vi "probe pulse.vi"(0 "Absolute start time (ms)":dbl=62793.546 format="%.3f", 1 "Static input":T4(array[cluster])=[{"Times"=[954.0, 1000.1, 6500.0], "Voltages"=[-0.05, -0.95, 2.0], "Enable Ch"=TRUE, "Hinge Points"=3}, {"Times"=[944.0, 994.0, 1000.0], "Voltages"=[-1.0, 1.65, -1.0], "Enable Ch"=TRUE, "Hinge Points"=3}, {"Times"=[944.0, 994.0, 1000.0], "Voltages"=[0.0, 0.4, -1.0], "Enable Ch"=TRUE, "Hinge Points"=3}, {"Times"=[944.0, 994.0, 1000.0], "Voltages"=[4.0, 0.65, -1.0], "Enable Ch"=TRUE, "Hinge Points"=3}, {"Times"=[992.0, 1000.6, 62293.246, 62294.046], "Voltages"=[0.0, 2.7, -0.8, 0.0], "Enable Ch"=TRUE, "Hinge Points"=4}, {"Times"=[1000.6, 1011.1], "Voltages"=[0.3, 3.0], "Enable Ch"=TRUE, "Hinge Points"=2}, {"Times"=[], "Voltages"=[], "Enable Ch"=TRUE, "Hinge Points"=0}, {"Times"=[62288.546], "Voltages"=[0.0], "Enable Ch"=TRUE, "Hinge Points"=1}, {"Times"=[944.0, 994.0, 1000.1, 1004.1, 6500.0], "Voltages"=[0.1635, 0.04, -0.625, 0.0, 1.0], "Enable Ch"=TRUE, "Hinge Points"=5}, {"Times"=[994.0, 1000.0, 1001.0, 1003.1, 1203.1, 1208.1, 1213.1, 1218.1, 1223.1, 1228.1, 1233.1, 1238.1, 1243.1, 1248.1, 1253.1, 1258.1, 1263.1, 1268.1, 1273.1, 1278.1, 1283.1, 1288.1, 1293.1, 1298.1, 1303.1, 1308.1, 1313.1, 1318.1, 1323.1, 1328.1, 1333.1, 1338.1, 1343.1, 1348.1, 1353.1, 1358.1, 1363.1, 1368.1, 1373.1, 1378.1, 1383.1, 1388.1, 1393.1, 1398.1, 1403.1, 1408.1, 1413.1, 1418.1, 1423.1, 1428.1, 1433.1, 1438.1, 1443.1, 1448.1, 1453.1, 1458.1, 1463.1, 1468.1, 1473.1, 1478.1, 1483.1, 1488.1, 1493.1, 1498.1, 1503.1, 1508.1, 1513.1, 1518.1, 1523.1, 1528.1, 1533.1, 1538.1, 1543.1, 1548.1, 1553.1, 1558.1, 1563.1, 1568.1, 1573.1, 1578.1, 1583.1, 1588.1, 1593.1, 1598.1, 1603.1, 1608.1, 1613.1, 1618.1, 1623.1, 1628.1, 1633.1, 1638.1, 1643.1, 1648.1, 1653.1, 1658.1, 1663.1, 1668.1, 1673.1, 1678.1, 1683.1, 1688.1, 1693.1, 1698.1, 1703.1, 5499.9], "Voltages"=[-1.0, -10.0, 0.0, 1.8, 1.8, 1.844, 1.8880000000000001, 1.932, 1.976, 2.02, 2.064, 2.108, 2.152, 2.196, 2.24, 2.2840000000000003, 2.3280000000000003, 2.372, 2.4160000000000004, 2.46, 2.504, 2.548, 2.592, 2.636, 2.68, 2.724, 2.7680000000000002, 2.8120000000000003, 2.856, 2.9000000000000004, 2.944, 2.9880000000000004, 3.032, 3.076, 3.12, 3.164, 3.208, 3.2520000000000002, 3.2960000000000003, 3.3400000000000003, 3.3840000000000003, 3.428, 3.4720000000000004, 3.516, 3.5600000000000005, 3.604, 3.648, 3.692, 3.736, 3.7800000000000002, 3.824, 3.8680000000000003, 3.912, 3.9560000000000004, 4.0, 4.0440000000000005, 4.088, 4.132000000000001, 4.176, 4.220000000000001, 4.264, 4.308000000000001, 4.352, 4.396, 4.44, 4.484, 4.5280000000000005, 4.572, 4.6160000000000005, 4.66, 4.704000000000001, 4.748, 4.792000000000001, 4.836, 4.880000000000001, 4.924, 4.968, 5.0120000000000005, 5.056, 5.1000000000000005, 5.144, 5.188000000000001, 5.232, 5.276000000000001, 5.32, 5.364000000000001, 5.408, 5.452000000000001, 5.496, 5.54, 5.5840000000000005, 5.628, 5.672000000000001, 5.716, 5.760000000000001, 5.804, 5.848, 5.892, 5.936, 5.98, 6.024, 6.0680000000000005, 6.112, 6.156000000000001, 6.2, -1.0], "Enable Ch"=TRUE, "Hinge Points"=106}, {"Times"=[1001.0, 978.1, 1008.1, 1183.1, 1188.1, 1193.1, 1198.1, 1203.1, 1208.1, 1213.1, 1218.1, 1223.1, 1228.1, 1233.1, 1238.1, 1243.1, 1248.1, 1253.1, 1258.1, 1263.1, 1268.1, 1273.1, 1278.1, 1283.1, 1288.1, 1293.1, 1298.1, 1303.1, 1308.1, 1313.1, 1318.1, 1323.1, 1328.1, 1333.1, 1338.1, 1343.1, 1348.1, 1353.1, 1358.1, 1363.1, 1368.1, 1373.1, 1378.1, 1383.1, 1388.1, 1393.1, 1398.1, 1403.1, 1408.1, 1413.1, 1418.1, 1423.1, 1428.1, 1433.1, 1438.1, 1443.1, 1448.1, 1453.1, 1458.1, 1463.1, 1468.1, 1473.1, 1478.1, 1483.1, 1488.1, 1493.1, 1498.1, 1503.1, 1508.1, 1513.1, 1518.1, 1523.1, 1528.1, 1533.1, 1538.1, 1543.1, 1548.1, 1553.1, 1558.1, 1563.1, 1568.1, 1573.1, 1578.1, 1583.1, 1588.1, 1593.1, 1598.1, 1603.1, 1608.1, 1613.1, 1618.1, 1623.1, 1628.1, 1633.1, 1638.1, 1643.1, 1648.1, 1653.1, 1658.1, 1663.1, 1668.1, 1673.1, 1678.1, 1683.1, 5505.0, 62273.546], "Voltages"=[-0.4, -2.5, -0.78, -0.78, -0.7989, -0.8178000000000001, -0.8367, -0.8556, -0.8745, -0.8934, -0.9123, -0.9312, -0.9501000000000001, -0.9690000000000001, -0.9879, -1.0068000000000001, -1.0257, -1.0446, -1.0635, -1.0824, -1.1013000000000002, -1.1202, -1.1391, -1.158, -1.1769, -1.1958, -1.2147000000000001, -1.2336, -1.2525, -1.2714, -1.2903, -1.3092000000000001, -1.3281, -1.347, -1.3659, -1.3848, -1.4037000000000002, -1.4226, -1.4415, -1.4604, -1.4793, -1.4982, -1.5171000000000001, -1.536, -1.5549, -1.5738, -1.5927, -1.6116000000000001, -1.6305, -1.6494, -1.6683, -1.6872, -1.7061000000000002, -1.725, -1.7439, -1.7628, -1.7817, -1.8006, -1.8195000000000001, -1.8384, -1.8573, -1.8762, -1.8951, -1.914, -1.9329, -1.9518, -1.9707000000000001, -1.9896, -2.0084999999999997, -2.0274, -2.0463, -2.0652, -2.0841000000000003, -2.1029999999999998, -2.1219, -2.1408, -2.1597, -2.1786000000000003, -2.1975, -2.2164, -2.2353, -2.2542, -2.2731000000000003, -2.292, -2.3109, -2.3298, -2.3487, -2.3676000000000004, -2.3865, -2.4054, -2.4243, -2.4432, -2.4621, -2.481, -2.4999000000000002, -2.5187999999999997, -2.5377, -2.5566, -2.5755, -2.5944000000000003, -2.6132999999999997, -2.6322, -2.6511, -2.67, -1.5, -1.5], "Enable Ch"=TRUE, "Hinge Points"=106}, {"Times"=[944.0, 994.0, 1000.6, 62291.546, 62294.046], "Voltages"=[0.15, 0.2, 2.5, -0.4, 0.0], "Enable Ch"=TRUE, "Hinge Points"=5}, {"Times"=[5500.0, 62273.546, 62273.548, 62273.55, 62273.552, 62273.554000000004, 62273.556000000004, 62273.558000000005, 62273.560000000005, 62273.562000000005, 62273.564, 62273.566, 62273.568, 62273.57, 62273.572, 62273.574, 62273.576, 62273.578, 62273.58, 62273.582, 62273.584, 62273.586], "Voltages"=[2.98, 2.98, 2.826, 2.672, 2.518, 2.364, 2.21, 2.056, 1.902, 1.748, 1.594, 1.44, 1.286, 1.1320000000000001, 0.9780000000000002, 0.8239999999999998, 0.6699999999999999, 0.516, 0.3620000000000001, 0.20800000000000018, 0.053999999999999826, -0.10000000000000009], "Enable Ch"=TRUE, "Hinge Points"=22}, {"Times"=[5500.0, 5600.0, 5609.0, 5618.0, 5627.0, 5636.0, 5645.0, 5654.0, 5663.0, 5672.0, 5681.0, 5690.0, 5699.0, 5708.0, 5717.0, 5726.0, 5735.0, 5744.0, 5753.0, 5762.0, 5771.0, 5780.0, 5789.0, 5798.0, 5807.0, 5816.0, 5825.0, 5834.0, 5843.0, 5852.0, 5861.0, 5870.0, 5879.0, 5888.0, 5897.0, 5906.0, 5915.0, 5924.0, 5933.0, 5942.0, 5951.0, 5960.0, 5969.0, 5978.0, 5987.0, 5996.0, 6005.0, 6014.0, 6023.0, 6032.0, 6041.0, 6050.0, 6059.0, 6068.0, 6077.0, 6086.0, 6095.0, 6104.0, 6113.0, 6122.0, 6131.0, 6140.0, 6149.0, 6158.0, 6167.0, 6176.0, 6185.0, 6194.0, 6203.0, 6212.0, 6221.0, 6230.0, 6239.0, 6248.0, 6257.0, 6266.0, 6275.0, 6284.0, 6293.0, 6302.0, 6311.0, 6320.0, 6329.0, 6338.0, 6347.0, 6356.0, 6365.0, 6374.0, 6383.0, 6392.0, 6401.0, 6410.0, 6419.0, 6428.0, 6437.0, 6446.0, 6455.0, 6464.0, 6473.0, 6482.0, 6491.0, 6500.0, 62273.546, 62303.546], "Voltages"=[0.5, 0.5, 0.5067, 0.5134, 0.5201, 0.5268, 0.5335, 0.5402, 0.5468999999999999, 0.5536, 0.5603, 0.567, 0.5737, 0.5804, 0.5871, 0.5938, 0.6005, 0.6072, 0.6139, 0.6206, 0.6273, 0.634, 0.6407, 0.6474, 0.6541, 0.6608, 0.6675, 0.6742, 0.6809, 0.6876, 0.6942999999999999, 0.701, 0.7077, 0.7143999999999999, 0.7211, 0.7278, 0.7344999999999999, 0.7412, 0.7479, 0.7545999999999999, 0.7613, 0.768, 0.7746999999999999, 0.7814, 0.7881, 0.7948, 0.8015, 0.8082, 0.8149, 0.8216, 0.8283, 0.835, 0.8416999999999999, 0.8484, 0.8551, 0.8617999999999999, 0.8684999999999999, 0.8752, 0.8818999999999999, 0.8886, 0.8953, 0.9019999999999999, 0.9087, 0.9154, 0.9220999999999999, 0.9288, 0.9355, 0.9421999999999999, 0.9489, 0.9556, 0.9622999999999999, 0.969, 0.9757, 0.9823999999999999, 0.9891, 0.9958, 1.0025, 1.0091999999999999, 1.0158999999999998, 1.0226, 1.0293, 1.036, 1.0427, 1.0493999999999999, 1.0560999999999998, 1.0628, 1.0695, 1.0762, 1.0829, 1.0896, 1.0962999999999998, 1.103, 1.1097, 1.1164, 1.1231, 1.1298, 1.1364999999999998, 1.1432, 1.1499, 1.1566, 1.1633, 1.17, -1.0, 0.0], "Enable Ch"=TRUE, "Hinge Points"=104}, {"Times"=[1000.6, 62283.546, 62295.546], "Voltages"=[1.3, -2.175, 0.0], "Enable Ch"=TRUE, "Hinge Points"=3}, {"Times"=[62283.546], "Voltages"=[-1.0], "Enable Ch"=TRUE, "Hinge Points"=1}] {"Voltages" format="%.2f"; "Times" format="%.2f"}, 2 "Input":i32[][](array[numeric])=[[-1000, 0, 5, 0], [-1000, 0, 8, 0], [-1000, 0, 8, 0], [-1000, 0, 8, 1], [-1000, 0, 9, 0], [-1000, 0, 10, 0], [-1000, 0, 10, 1], [-1000, 0, 13, 0], [-1000, 0, 13, 1], [944000, 3, 14, 1], [944000, 3, 14, 1], [944000, 3, 14, 1], [944000, 3, 15, 1], [944000, 3, 15, 1], [944001, 3, 14, 0], [944001, 3, 14, 0], [944001, 3, 14, 0], [944001, 3, 15, 0], [944001, 3, 15, 0], [951100, 0, 6, 1], [951100, 1, 7, 1], [954000, 3, 14, 1], [954001, 3, 14, 0], [978100, 3, 15, 1], [978101, 3, 15, 0], [992000, 3, 14, 1], [992001, 3, 14, 0], [994000, 3, 14, 1], [994000, 3, 14, 1], [994000, 3, 14, 1], [994000, 3, 15, 1], [994000, 3, 15, 1], [994000, 3, 15, 1], [994001, 3, 14, 0], [994001, 3, 14, 0], [994001, 3, 14, 0], [994001, 3, 15, 0], [994001, 3, 15, 0], [994001, 3, 15, 0], [998300, 0, 2, 0], [998300, 0, 4, 0], [998400, 0, 8, 1], [998400, 0, 9, 1], [999000, 0, 3, 0], [999100, 1, 9, 1], [1000000, 0, 10, 0], [1000000, 1, 0, 0], [1000000, 3, 14, 1], [1000000, 3, 14, 1], [1000000, 3, 14, 1], [1000000, 3, 15, 1], [1000001, 3, 14, 0], [1000001, 3, 14, 0], [1000001, 3, 14, 0], [1000001, 3, 15, 0], [1000100, 3, 14, 1], [1000100, 3, 15, 1], [1000101, 3, 14, 0], [1000101, 3, 15, 0], [1000600, 3, 14, 1], [1000600, 3, 14, 1], [1000600, 3, 15, 1], [1000600, 3, 15, 1], [1000601, 3, 14, 0], [1000601, 3, 14, 0], [1000601, 3, 15, 0], [1000601, 3, 15, 0], [1001000, 3, 15, 1], [1001000, 3, 15, 1], [1001001, 3, 15, 0], [1001001, 3, 15, 0], [1001100, 0, 5, 1], [1001100, 0, 10, 1], [1001100, 1, 1, 1], [1002100, 1, 1, 0], [1002100, 1, 9, 0], [1002600, 0, 5, 0], [1003100, 0, 8, 0], [1003100, 0, 9, 0], [1003100, 1, 0, 1], [1003100, 3, 15, 1], [1003101, 3, 15, 0], [1004100, 0, 6, 0], [1004100, 0, 10, 0], [1004100, 1, 7, 0], [1004100, 3, 15, 1], [1004101, 3, 15, 0], [1008100, 3, 15, 1], [1008101, 3, 15, 0], [1011100, 3, 14, 1], [1011101, 3, 14, 0], [1183100, 3, 15, 1], [1183101, 3, 15, 0], [1188100, 3, 15, 1], [1188101, 3, 15, 0], [1193100, 3, 15, 1], [1193101, 3, 15, 0], [1198100, 3, 15, 1], [1198101, 3, 15, 0], [1203100, 3, 15, 1], [1203100, 3, 15, 1], [1203101, 3, 15, 0], [1203101, 3, 15, 0], [1208100, 3, 15, 1], [1208100, 3, 15, 1], [1208101, 3, 15, 0], [1208101, 3, 15, 0], [1213100, 3, 15, 1], [1213100, 3, 15, 1], [1213101, 3, 15, 0], [1213101, 3, 15, 0], [1218100, 3, 15, 1], [1218100, 3, 15, 1], [1218101, 3, 15, 0], [1218101, 3, 15, 0], [1223100, 3, 15, 1], [1223100, 3, 15, 1], [1223101, 3, 15, 0], [1223101, 3, 15, 0], [1228100, 3, 15, 1], [1228100, 3, 15, 1], [1228101, 3, 15, 0], [1228101, 3, 15, 0], [1233100, 3, 15, 1], [1233100, 3, 15, 1], [1233101, 3, 15, 0], [1233101, 3, 15, 0], [1238100, 3, 15, 1], [1238100, 3, 15, 1], [1238101, 3, 15, 0], [1238101, 3, 15, 0], [1243100, 3, 15, 1], [1243100, 3, 15, 1], [1243101, 3, 15, 0], [1243101, 3, 15, 0], [1248100, 3, 15, 1], [1248100, 3, 15, 1], [1248101, 3, 15, 0], [1248101, 3, 15, 0], [1253100, 3, 15, 1], [1253100, 3, 15, 1], [1253101, 3, 15, 0], [1253101, 3, 15, 0], [1258100, 3, 15, 1], [1258100, 3, 15, 1], [1258101, 3, 15, 0], [1258101, 3, 15, 0], [1263100, 3, 15, 1], [1263100, 3, 15, 1], [1263101, 3, 15, 0], [1263101, 3, 15, 0], [1268100, 3, 15, 1], [1268100, 3, 15, 1], [1268101, 3, 15, 0], [1268101, 3, 15, 0], [1273100, 3, 15, 1], [1273100, 3, 15, 1], [1273101, 3, 15, 0], [1273101, 3, 15, 0], [1278100, 3, 15, 1], [1278100, 3, 15, 1], [1278101, 3, 15, 0], [1278101, 3, 15, 0], [1283100, 3, 15, 1], [1283100, 3, 15, 1], [1283101, 3, 15, 0], [1283101, 3, 15, 0], [1288100, 3, 15, 1], [1288100, 3, 15, 1], [1288101, 3, 15, 0], [1288101, 3, 15, 0], [1293100, 3, 15, 1], [1293100, 3, 15, 1], [1293101, 3, 15, 0], [1293101, 3, 15, 0], [1298100, 3, 15, 1], [1298100, 3, 15, 1], [1298101, 3, 15, 0], [1298101, 3, 15, 0], [1303100, 3, 15, 1], [1303100, 3, 15, 1], [1303101, 3, 15, 0], [1303101, 3, 15, 0], [1308100, 3, 15, 1], [1308100, 3, 15, 1], [1308101, 3, 15, 0], [1308101, 3, 15, 0], [1313100, 3, 15, 1], [1313100, 3, 15, 1], [1313101, 3, 15, 0], [1313101, 3, 15, 0], [1318100, 3, 15, 1], [1318100, 3, 15, 1], [1318101, 3, 15, 0], [1318101, 3, 15, 0], [1323100, 3, 15, 1], [1323100, 3, 15, 1], [1323101, 3, 15, 0], [1323101, 3, 15, 0], [1328100, 3, 15, 1], [1328100, 3, 15, 1], [1328101, 3, 15, 0], [1328101, 3, 15, 0], [1333100, 3, 15, 1], [1333100, 3, 15, 1], [1333101, 3, 15, 0], [1333101, 3, 15, 0], [1338100, 3, 15, 1], [1338100, 3, 15, 1], [1338101, 3, 15, 0], [1338101, 3, 15, 0], [1343100, 3, 15, 1], [1343100, 3, 15, 1], [1343101, 3, 15, 0], [1343101, 3, 15, 0], [1348100, 3, 15, 1], [1348100, 3, 15, 1], [1348101, 3, 15, 0], [1348101, 3, 15, 0], [1353100, 3, 15, 1], [1353100, 3, 15, 1], [1353101, 3, 15, 0], [1353101, 3, 15, 0], [1358100, 3, 15, 1], [1358100, 3, 15, 1], [1358101, 3, 15, 0], [1358101, 3, 15, 0], [1363100, 3, 15, 1], [1363100, 3, 15, 1], [1363101, 3, 15, 0], [1363101, 3, 15, 0], [1368100, 3, 15, 1], [1368100, 3, 15, 1], [1368101, 3, 15, 0], [1368101, 3, 15, 0], [1373100, 3, 15, 1], [1373100, 3, 15, 1], [1373101, 3, 15, 0], [1373101, 3, 15, 0], [1378100, 3, 15, 1], [1378100, 3, 15, 1], [1378101, 3, 15, 0], [1378101, 3, 15, 0], [1383100, 3, 15, 1], [1383100, 3, 15, 1], [1383101, 3, 15, 0], [1383101, 3, 15, 0], [1388100, 3, 15, 1], [1388100, 3, 15, 1], [1388101, 3, 15, 0], [1388101, 3, 15, 0], [1393100, 3, 15, 1], [1393100, 3, 15, 1], [1393101, 3, 15, 0], [1393101, 3, 15, 0], [1398100, 3, 15, 1], [1398100, 3, 15, 1], [1398101, 3, 15, 0], [1398101, 3, 15, 0], [1403100, 3, 15, 1], [1403100, 3, 15, 1], [1403101, 3, 15, 0], [1403101, 3, 15, 0], [1408100, 3, 15, 1], [1408100, 3, 15, 1], [1408101, 3, 15, 0], [1408101, 3, 15, 0], [1413100, 3, 15, 1], [1413100, 3, 15, 1], [1413101, 3, 15, 0], [1413101, 3, 15, 0], [1418100, 3, 15, 1], [1418100, 3, 15, 1], [1418101, 3, 15, 0], [1418101, 3, 15, 0], [1423100, 3, 15, 1], [1423100, 3, 15, 1], [1423101, 3, 15, 0], [1423101, 3, 15, 0], [1428100, 3, 15, 1], [1428100, 3, 15, 1], [1428101, 3, 15, 0], [1428101, 3, 15, 0], [1433100, 3, 15, 1], [1433100, 3, 15, 1], [1433101, 3, 15, 0], [1433101, 3, 15, 0], [1438100, 3, 15, 1], [1438100, 3, 15, 1], [1438101, 3, 15, 0], [1438101, 3, 15, 0], [1443100, 3, 15, 1], [1443100, 3, 15, 1], [1443101, 3, 15, 0], [1443101, 3, 15, 0], [1448100, 3, 15, 1], [1448100, 3, 15, 1], [1448101, 3, 15, 0], [1448101, 3, 15, 0], [1453100, 3, 15, 1], [1453100, 3, 15, 1], [1453101, 3, 15, 0], [1453101, 3, 15, 0], [1458100, 3, 15, 1], [1458100, 3, 15, 1], [1458101, 3, 15, 0], [1458101, 3, 15, 0], [1463100, 3, 15, 1], [1463100, 3, 15, 1], [1463101, 3, 15, 0], [1463101, 3, 15, 0], [1468100, 3, 15, 1], [1468100, 3, 15, 1], [1468101, 3, 15, 0], [1468101, 3, 15, 0], [1473100, 3, 15, 1], [1473100, 3, 15, 1], [1473101, 3, 15, 0], [1473101, 3, 15, 0], [1478100, 3, 15, 1], [1478100, 3, 15, 1], [1478101, 3, 15, 0], [1478101, 3, 15, 0], [1483100, 3, 15, 1], [1483100, 3, 15, 1], [1483101, 3, 15, 0], [1483101, 3, 15, 0], [1488100, 3, 15, 1], [1488100, 3, 15, 1], [1488101, 3, 15, 0], [1488101, 3, 15, 0], [1493100, 3, 15, 1], [1493100, 3, 15, 1], [1493101, 3, 15, 0], [1493101, 3, 15, 0], [1498100, 3, 15, 1], [1498100, 3, 15, 1], [1498101, 3, 15, 0], [1498101, 3, 15, 0], [1500000, 1, 3, 1], [1503100, 3, 15, 1], [1503100, 3, 15, 1], [1503101, 3, 15, 0], [1503101, 3, 15, 0], [1508100, 3, 15, 1], [1508100, 3, 15, 1], [1508101, 3, 15, 0], [1508101, 3, 15, 0], [1513100, 3, 15, 1], [1513100, 3, 15, 1], [1513101, 3, 15, 0], [1513101, 3, 15, 0], [1518100, 3, 15, 1], [1518100, 3, 15, 1], [1518101, 3, 15, 0], [1518101, 3, 15, 0], [1523100, 3, 15, 1], [1523100, 3, 15, 1], [1523101, 3, 15, 0], [1523101, 3, 15, 0], [1528100, 3, 15, 1], [1528100, 3, 15, 1], [1528101, 3, 15, 0], [1528101, 3, 15, 0], [1533100, 3, 15, 1], [1533100, 3, 15, 1], [1533101, 3, 15, 0], [1533101, 3, 15, 0], [1538100, 3, 15, 1], [1538100, 3, 15, 1], [1538101, 3, 15, 0], [1538101, 3, 15, 0], [1543100, 3, 15, 1], [1543100, 3, 15, 1], [1543101, 3, 15, 0], [1543101, 3, 15, 0], [1548100, 3, 15, 1], [1548100, 3, 15, 1], [1548101, 3, 15, 0], [1548101, 3, 15, 0], [1553100, 3, 15, 1], [1553100, 3, 15, 1], [1553101, 3, 15, 0], [1553101, 3, 15, 0], [1558100, 3, 15, 1], [1558100, 3, 15, 1], [1558101, 3, 15, 0], [1558101, 3, 15, 0], [1563100, 3, 15, 1], [1563100, 3, 15, 1], [1563101, 3, 15, 0], [1563101, 3, 15, 0], [1568100, 3, 15, 1], [1568100, 3, 15, 1], [1568101, 3, 15, 0], [1568101, 3, 15, 0], [1573100, 3, 15, 1], [1573100, 3, 15, 1], [1573101, 3, 15, 0], [1573101, 3, 15, 0], [1578100, 3, 15, 1], [1578100, 3, 15, 1], [1578101, 3, 15, 0], [1578101, 3, 15, 0], [1583100, 3, 15, 1], [1583100, 3, 15, 1], [1583101, 3, 15, 0], [1583101, 3, 15, 0], [1588100, 3, 15, 1], [1588100, 3, 15, 1], [1588101, 3, 15, 0], [1588101, 3, 15, 0], [1593100, 3, 15, 1], [1593100, 3, 15, 1], [1593101, 3, 15, 0], [1593101, 3, 15, 0], [1598100, 3, 15, 1], [1598100, 3, 15, 1], [1598101, 3, 15, 0], [1598101, 3, 15, 0], [1603100, 3, 15, 1], [1603100, 3, 15, 1], [1603101, 3, 15, 0], [1603101, 3, 15, 0], [1608100, 3, 15, 1], [1608100, 3, 15, 1], [1608101, 3, 15, 0], [1608101, 3, 15, 0], [1613100, 3, 15, 1], [1613100, 3, 15, 1], [1613101, 3, 15, 0], [1613101, 3, 15, 0], [1618100, 3, 15, 1], [1618100, 3, 15, 1], [1618101, 3, 15, 0], [1618101, 3, 15, 0], [1623100, 3, 15, 1], [1623100, 3, 15, 1], [1623101, 3, 15, 0], [1623101, 3, 15, 0], [1628100, 3, 15, 1], [1628100, 3, 15, 1], [1628101, 3, 15, 0], [1628101, 3, 15, 0], [1633100, 3, 15, 1], [1633100, 3, 15, 1], [1633101, 3, 15, 0], [1633101, 3, 15, 0], [1638100, 3, 15, 1], [1638100, 3, 15, 1], [1638101, 3, 15, 0], [1638101, 3, 15, 0], [1643100, 3, 15, 1], [1643100, 3, 15, 1], [1643101, 3, 15, 0], [1643101, 3, 15, 0], [1648100, 3, 15, 1], [1648100, 3, 15, 1], [1648101, 3, 15, 0], [1648101, 3, 15, 0], [1653100, 3, 15, 1], [1653100, 3, 15, 1], [1653101, 3, 15, 0], [1653101, 3, 15, 0], [1658100, 3, 15, 1], [1658100, 3, 15, 1], [1658101, 3, 15, 0], [1658101, 3, 15, 0], [1663100, 3, 15, 1], [1663100, 3, 15, 1], [1663101, 3, 15, 0], [1663101, 3, 15, 0], [1668100, 3, 15, 1], [1668100, 3, 15, 1], [1668101, 3, 15, 0], [1668101, 3, 15, 0], [1673100, 3, 15, 1], [1673100, 3, 15, 1], [1673101, 3, 15, 0], [1673101, 3, 15, 0], [1678100, 3, 15, 1], [1678100, 3, 15, 1], [1678101, 3, 15, 0], [1678101, 3, 15, 0], [1683100, 3, 15, 1], [1683100, 3, 15, 1], [1683101, 3, 15, 0], [1683101, 3, 15, 0], [1688100, 3, 15, 1], [1688101, 3, 15, 0], [1693100, 3, 15, 1], [1693101, 3, 15, 0], [1698100, 3, 15, 1], [1698101, 3, 15, 0], [1703100, 3, 15, 1], [1703101, 3, 15, 0], [5499900, 3, 15, 1], [5499901, 3, 15, 0], [5500000, 1, 14, 1], [5500000, 1, 15, 1], [5500000, 3, 15, 1], [5500000, 3, 15, 1], [5500001, 3, 15, 0], [5500001, 3, 15, 0], [5505000, 3, 15, 1], [5505001, 3, 15, 0], [5600000, 3, 15, 1], [5600001, 3, 15, 0], [5609000, 3, 15, 1], [5609001, 3, 15, 0], [5618000, 3, 15, 1], [5618001, 3, 15, 0], [5627000, 3, 15, 1], [5627001, 3, 15, 0], [5636000, 3, 15, 1], [5636001, 3, 15, 0], [5645000, 3, 15, 1], [5645001, 3, 15, 0], [5654000, 3, 15, 1], [5654001, 3, 15, 0], [5663000, 3, 15, 1], [5663001, 3, 15, 0], [5672000, 3, 15, 1], [5672001, 3, 15, 0], [5681000, 3, 15, 1], [5681001, 3, 15, 0], [5690000, 3, 15, 1], [5690001, 3, 15, 0], [5699000, 3, 15, 1], [5699001, 3, 15, 0], [5708000, 3, 15, 1], [5708001, 3, 15, 0], [5717000, 3, 15, 1], [5717001, 3, 15, 0], [5726000, 3, 15, 1], [5726001, 3, 15, 0], [5735000, 3, 15, 1], [5735001, 3, 15, 0], [5744000, 3, 15, 1], [5744001, 3, 15, 0], [5753000, 3, 15, 1], [5753001, 3, 15, 0], [5762000, 3, 15, 1], [5762001, 3, 15, 0], [5771000, 3, 15, 1], [5771001, 3, 15, 0], [5780000, 3, 15, 1], [5780001, 3, 15, 0], [5789000, 3, 15, 1], [5789001, 3, 15, 0], [5798000, 3, 15, 1], [5798001, 3, 15, 0], [5807000, 3, 15, 1], [5807001, 3, 15, 0], [5816000, 3, 15, 1], [5816001, 3, 15, 0], [5825000, 3, 15, 1], [5825001, 3, 15, 0], [5834000, 3, 15, 1], [5834001, 3, 15, 0], [5843000, 3, 15, 1], [5843001, 3, 15, 0], [5852000, 3, 15, 1], [5852001, 3, 15, 0], [5861000, 3, 15, 1], [5861001, 3, 15, 0], [5870000, 3, 15, 1], [5870001, 3, 15, 0], [5879000, 3, 15, 1], [5879001, 3, 15, 0], [5888000, 3, 15, 1], [5888001, 3, 15, 0], [5897000, 3, 15, 1], [5897001, 3, 15, 0], [5906000, 3, 15, 1], [5906001, 3, 15, 0], [5915000, 3, 15, 1], [5915001, 3, 15, 0], [5924000, 3, 15, 1], [5924001, 3, 15, 0], [5933000, 3, 15, 1], [5933001, 3, 15, 0], [5942000, 3, 15, 1], [5942001, 3, 15, 0], [5951000, 3, 15, 1], [5951001, 3, 15, 0], [5960000, 3, 15, 1], [5960001, 3, 15, 0], [5969000, 3, 15, 1], [5969001, 3, 15, 0], [5978000, 3, 15, 1], [5978001, 3, 15, 0], [5987000, 3, 15, 1], [5987001, 3, 15, 0], [5996000, 3, 15, 1], [5996001, 3, 15, 0], [6005000, 3, 15, 1], [6005001, 3, 15, 0], [6014000, 3, 15, 1], [6014001, 3, 15, 0], [6023000, 3, 15, 1], [6023001, 3, 15, 0], [6032000, 3, 15, 1], [6032001, 3, 15, 0], [6041000, 3, 15, 1], [6041001, 3, 15, 0], [6050000, 3, 15, 1], [6050001, 3, 15, 0], [6059000, 3, 15, 1], [6059001, 3, 15, 0], [6068000, 3, 15, 1], [6068001, 3, 15, 0], [6077000, 3, 15, 1], [6077001, 3, 15, 0], [6086000, 3, 15, 1], [6086001, 3, 15, 0], [6095000, 3, 15, 1], [6095001, 3, 15, 0], [6104000, 3, 15, 1], [6104001, 3, 15, 0], [6113000, 3, 15, 1], [6113001, 3, 15, 0], [6122000, 3, 15, 1], [6122001, 3, 15, 0], [6131000, 3, 15, 1], [6131001, 3, 15, 0], [6140000, 3, 15, 1], [6140001, 3, 15, 0], [6149000, 3, 15, 1], [6149001, 3, 15, 0], [6158000, 3, 15, 1], [6158001, 3, 15, 0], [6167000, 3, 15, 1], [6167001, 3, 15, 0], [6176000, 3, 15, 1], [6176001, 3, 15, 0], [6185000, 3, 15, 1], [6185001, 3, 15, 0], [6194000, 3, 15, 1], [6194001, 3, 15, 0], [6203000, 3, 15, 1], [6203001, 3, 15, 0], [6212000, 3, 15, 1], [6212001, 3, 15, 0], [6221000, 3, 15, 1], [6221001, 3, 15, 0], [6230000, 3, 15, 1], [6230001, 3, 15, 0], [6239000, 3, 15, 1], [6239001, 3, 15, 0], [6248000, 3, 15, 1], [6248001, 3, 15, 0], [6257000, 3, 15, 1], [6257001, 3, 15, 0], [6266000, 3, 15, 1], [6266001, 3, 15, 0], [6275000, 3, 15, 1], [6275001, 3, 15, 0], [6284000, 3, 15, 1], [6284001, 3, 15, 0], [6293000, 3, 15, 1], [6293001, 3, 15, 0], [6302000, 3, 15, 1], [6302001, 3, 15, 0], [6311000, 3, 15, 1], [6311001, 3, 15, 0], [6320000, 3, 15, 1], [6320001, 3, 15, 0], [6329000, 3, 15, 1], [6329001, 3, 15, 0], [6338000, 3, 15, 1], [6338001, 3, 15, 0], [6347000, 3, 15, 1], [6347001, 3, 15, 0], [6356000, 3, 15, 1], [6356001, 3, 15, 0], [6365000, 3, 15, 1], [6365001, 3, 15, 0], [6374000, 3, 15, 1], [6374001, 3, 15, 0], [6383000, 3, 15, 1], [6383001, 3, 15, 0], [6392000, 3, 15, 1], [6392001, 3, 15, 0], [6401000, 3, 15, 1], [6401001, 3, 15, 0], [6410000, 3, 15, 1], [6410001, 3, 15, 0], [6419000, 3, 15, 1], [6419001, 3, 15, 0], [6428000, 3, 15, 1], [6428001, 3, 15, 0], [6437000, 3, 15, 1], [6437001, 3, 15, 0], [6446000, 3, 15, 1], [6446001, 3, 15, 0], [6455000, 3, 15, 1], [6455001, 3, 15, 0], [6464000, 3, 15, 1], [6464001, 3, 15, 0], [6473000, 3, 15, 1], [6473001, 3, 15, 0], [6482000, 3, 15, 1], [6482001, 3, 15, 0], [6491000, 3, 15, 1], [6491001, 3, 15, 0], [6500000, 3, 14, 1], [6500000, 3, 15, 1], [6500000, 3, 15, 1], [6500001, 3, 14, 0], [6500001, 3, 15, 0], [6500001, 3, 15, 0], [7500000, 1, 0, 0], [7500000, 1, 3, 0], [62173546, 1, 14, 0], [62223546, 1, 8, 1], [62272746, 1, 9, 1], [62273546, 3, 15, 1], [62273546, 3, 15, 1], [62273546, 3, 15, 1], [62273547, 3, 15, 0], [62273547, 3, 15, 0], [62273547, 3, 15, 0], [62273548, 3, 15, 1], [62273549, 3, 15, 0], [62273550, 3, 15, 1], [62273551, 3, 15, 0], [62273552, 3, 15, 1], [62273553, 3, 15, 0], [62273554, 3, 15, 1], [62273555, 3, 15, 0], [62273556, 3, 15, 1], [62273557, 3, 15, 0], [62273558, 3, 15, 1], [62273559, 3, 15, 0], [62273560, 3, 15, 1], [62273561, 3, 15, 0], [62273562, 3, 15, 1], [62273563, 3, 15, 0], [62273564, 3, 15, 1], [62273565, 3, 15, 0], [62273566, 3, 15, 1], [62273567, 3, 15, 0], [62273568, 3, 15, 1], [62273569, 3, 15, 0], [62273570, 3, 15, 1], [62273571, 3, 15, 0], [62273572, 3, 15, 1], [62273573, 3, 15, 0], [62273574, 3, 15, 1], [62273575, 3, 15, 0], [62273576, 3, 15, 1], [62273577, 3, 15, 0], [62273578, 3, 15, 1], [62273579, 3, 15, 0], [62273580, 3, 15, 1], [62273581, 3, 15, 0], [62273582, 3, 15, 1], [62273583, 3, 15, 0], [62273584, 3, 15, 1], [62273585, 3, 15, 0], [62273586, 3, 15, 1], [62273587, 3, 15, 0], [62283546, 3, 15, 1], [62283546, 3, 15, 1], [62283547, 3, 15, 0], [62283547, 3, 15, 0], [62287546, 0, 1, 1], [62288546, 3, 14, 1], [62288547, 3, 14, 0], [62289546, 0, 7, 1], [62290546, 1, 14, 1], [62291546, 3, 15, 1], [62291547, 3, 15, 0], [62293246, 3, 14, 1], [62293247, 3, 14, 0], [62293346, 0, 12, 1], [62293446, 1, 7, 1], [62293546, 0, 1, 0], [62293546, 0, 12, 0], [62293546, 0, 15, 1], [62293546, 1, 1, 1], [62293646, 0, 7, 0], [62293646, 0, 15, 0], [62293646, 1, 1, 0], [62293646, 1, 7, 0], [62293646, 1, 14, 0], [62294046, 3, 14, 1], [62294046, 3, 15, 1], [62294047, 3, 14, 0], [62294047, 3, 15, 0], [62295546, 3, 15, 1], [62295547, 3, 15, 0], [62303546, 3, 15, 1], [62303547, 3, 15, 0], [62323546, 1, 9, 0], [62373546, 1, 15, 0]], 3 "GPIB Input":T1(array[cluster]) {"Module" items=["TTL high                                                                                 ", "TTL low                          ", "Camera Strobe                   ", "CMOT", "Defaults                           ", "Fluorescence pulse           ", "IP trap                         ", "Kinetics OD image          ", "Kinetics picture", "Kinetics probe pulse", "MOT light only                ", "MOT off                                   ", "MOT on                         ", "Move cart                      ", "OD image                     ", "Optical pumping          ", "Picture                             ", "Probe Pulse", "Quadrupole trap             ", "IP off", "Utility Module 02           ", "Utility Module 03           ", "Molasses          ", "Utility Module 04     ", "Utility Module 05     ", "Utility Module 06     ", "Utility Module 07     ", "Utility Module 08     ", "Utility Module 09     ", "Utility Module 10     ", "Static DAC", "GPIB"]; "Abs Start Time" format="%.3f"}, 4 "Do this?":bool=TRUE) -> (5 "Static output":T4(array[cluster])=[{"Times"=[954.0, 1000.1, 6500.0], "Voltages"=[-0.05, -0.95, 2.0], "Enable Ch"=TRUE, "Hinge Points"=3}, {"Times"=[944.0, 994.0, 1000.0], "Voltages"=[-1.0, 1.65, -1.0], "Enable Ch"=TRUE, "Hinge Points"=3}, {"Times"=[944.0, 994.0, 1000.0], "Voltages"=[0.0, 0.4, -1.0], "Enable Ch"=TRUE, "Hinge Points"=3}, {"Times"=[944.0, 994.0, 1000.0], "Voltages"=[4.0, 0.65, -1.0], "Enable Ch"=TRUE, "Hinge Points"=3}, {"Times"=[992.0, 1000.6, 62293.246, 62294.046, 62793.246, 62794.046], "Voltages"=[0.0, 2.7, -0.8, 0.0, -0.8, 0.0], "Enable Ch"=TRUE, "Hinge Points"=6}, {"Times"=[1000.6, 1011.1], "Voltages"=[0.3, 3.0], "Enable Ch"=TRUE, "Hinge Points"=2}, {"Times"=[], "Voltages"=[], "Enable Ch"=TRUE, "Hinge Points"=0}, {"Times"=[62288.546, 62788.546], "Voltages"=[0.0, 0.0], "Enable Ch"=TRUE, "Hinge Points"=2}, {"Times"=[944.0, 994.0, 1000.1, 1004.1, 6500.0], "Voltages"=[0.1635, 0.04, -0.625, 0.0, 1.0], "Enable Ch"=TRUE, "Hinge Points"=5}, {"Times"=[994.0, 1000.0, 1001.0, 1003.1, 1203.1, 1208.1, 1213.1, 1218.1, 1223.1, 1228.1, 1233.1, 1238.1, 1243.1, 1248.1, 1253.1, 1258.1, 1263.1, 1268.1, 1273.1, 1278.1, 1283.1, 1288.1, 1293.1, 1298.1, 1303.1, 1308.1, 1313.1, 1318.1, 1323.1, 1328.1, 1333.1, 1338.1, 1343.1, 1348.1, 1353.1, 1358.1, 1363.1, 1368.1, 1373.1, 1378.1, 1383.1, 1388.1, 1393.1, 1398.1, 1403.1, 1408.1, 1413.1, 1418.1, 1423.1, 1428.1, 1433.1, 1438.1, 1443.1, 1448.1, 1453.1, 1458.1, 1463.1, 1468.1, 1473.1, 1478.1, 1483.1, 1488.1, 1493.1, 1498.1, 1503.1, 1508.1, 1513.1, 1518.1, 1523.1, 1528.1, 1533.1, 1538.1, 1543.1, 1548.1, 1553.1, 1558.1, 1563.1, 1568.1, 1573.1, 1578.1, 1583.1, 1588.1, 1593.1, 1598.1, 1603.1, 1608.1, 1613.1, 1618.1, 1623.1, 1628.1, 1633.1, 1638.1, 1643.1, 1648.1, 1653.1, 1658.1, 1663.1, 1668.1, 1673.1, 1678.1, 1683.1, 1688.1, 1693.1, 1698.1, 1703.1, 5499.9], "Voltages"=[-1.0, -10.0, 0.0, 1.8, 1.8, 1.844, 1.8880000000000001, 1.932, 1.976, 2.02, 2.064, 2.108, 2.152, 2.196, 2.24, 2.2840000000000003, 2.3280000000000003, 2.372, 2.4160000000000004, 2.46, 2.504, 2.548, 2.592, 2.636, 2.68, 2.724, 2.7680000000000002, 2.8120000000000003, 2.856, 2.9000000000000004, 2.944, 2.9880000000000004, 3.032, 3.076, 3.12, 3.164, 3.208, 3.2520000000000002, 3.2960000000000003, 3.3400000000000003, 3.3840000000000003, 3.428, 3.4720000000000004, 3.516, 3.5600000000000005, 3.604, 3.648, 3.692, 3.736, 3.7800000000000002, 3.824, 3.8680000000000003, 3.912, 3.9560000000000004, 4.0, 4.0440000000000005, 4.088, 4.132000000000001, 4.176, 4.220000000000001, 4.264, 4.308000000000001, 4.352, 4.396, 4.44, 4.484, 4.5280000000000005, 4.572, 4.6160000000000005, 4.66, 4.704000000000001, 4.748, 4.792000000000001, 4.836, 4.880000000000001, 4.924, 4.968, 5.0120000000000005, 5.056, 5.1000000000000005, 5.144, 5.188000000000001, 5.232, 5.276000000000001, 5.32, 5.364000000000001, 5.408, 5.452000000000001, 5.496, 5.54, 5.5840000000000005, 5.628, 5.672000000000001, 5.716, 5.760000000000001, 5.804, 5.848, 5.892, 5.936, 5.98, 6.024, 6.0680000000000005, 6.112, 6.156000000000001, 6.2, -1.0], "Enable Ch"=TRUE, "Hinge Points"=106}, {"Times"=[1001.0, 978.1, 1008.1, 1183.1, 1188.1, 1193.1, 1198.1, 1203.1, 1208.1, 1213.1, 1218.1, 1223.1, 1228.1, 1233.1, 1238.1, 1243.1, 1248.1, 1253.1, 1258.1, 1263.1, 1268.1, 1273.1, 1278.1, 1283.1, 1288.1, 1293.1, 1298.1, 1303.1, 1308.1, 1313.1, 1318.1, 1323.1, 1328.1, 1333.1, 1338.1, 1343.1, 1348.1, 1353.1, 1358.1, 1363.1, 1368.1, 1373.1, 1378.1, 1383.1, 1388.1, 1393.1, 1398.1, 1403.1, 1408.1, 1413.1, 1418.1, 1423.1, 1428.1, 1433.1, 1438.1, 1443.1, 1448.1, 1453.1, 1458.1, 1463.1, 1468.1, 1473.1, 1478.1, 1483.1, 1488.1, 1493.1, 1498.1, 1503.1, 1508.1, 1513.1, 1518.1, 1523.1, 1528.1, 1533.1, 1538.1, 1543.1, 1548.1, 1553.1, 1558.1, 1563.1, 1568.1, 1573.1, 1578.1, 1583.1, 1588.1, 1593.1, 1598.1, 1603.1, 1608.1, 1613.1, 1618.1, 1623.1, 1628.1, 1633.1, 1638.1, 1643.1, 1648.1, 1653.1, 1658.1, 1663.1, 1668.1, 1673.1, 1678.1, 1683.1, 5505.0, 62273.546], "Voltages"=[-0.4, -2.5, -0.78, -0.78, -0.7989, -0.8178000000000001, -0.8367, -0.8556, -0.8745, -0.8934, -0.9123, -0.9312, -0.9501000000000001, -0.9690000000000001, -0.9879, -1.0068000000000001, -1.0257, -1.0446, -1.0635, -1.0824, -1.1013000000000002, -1.1202, -1.1391, -1.158, -1.1769, -1.1958, -1.2147000000000001, -1.2336, -1.2525, -1.2714, -1.2903, -1.3092000000000001, -1.3281, -1.347, -1.3659, -1.3848, -1.4037000000000002, -1.4226, -1.4415, -1.4604, -1.4793, -1.4982, -1.5171000000000001, -1.536, -1.5549, -1.5738, -1.5927, -1.6116000000000001, -1.6305, -1.6494, -1.6683, -1.6872, -1.7061000000000002, -1.725, -1.7439, -1.7628, -1.7817, -1.8006, -1.8195000000000001, -1.8384, -1.8573, -1.8762, -1.8951, -1.914, -1.9329, -1.9518, -1.9707000000000001, -1.9896, -2.0084999999999997, -2.0274, -2.0463, -2.0652, -2.0841000000000003, -2.1029999999999998, -2.1219, -2.1408, -2.1597, -2.1786000000000003, -2.1975, -2.2164, -2.2353, -2.2542, -2.2731000000000003, -2.292, -2.3109, -2.3298, -2.3487, -2.3676000000000004, -2.3865, -2.4054, -2.4243, -2.4432, -2.4621, -2.481, -2.4999000000000002, -2.5187999999999997, -2.5377, -2.5566, -2.5755, -2.5944000000000003, -2.6132999999999997, -2.6322, -2.6511, -2.67, -1.5, -1.5], "Enable Ch"=TRUE, "Hinge Points"=106}, {"Times"=[944.0, 994.0, 1000.6, 62291.546, 62294.046, 62791.546, 62794.046], "Voltages"=[0.15, 0.2, 2.5, -0.4, 0.0, -0.4, 0.0], "Enable Ch"=TRUE, "Hinge Points"=7}, {"Times"=[5500.0, 62273.546, 62273.548, 62273.55, 62273.552, 62273.554000000004, 62273.556000000004, 62273.558000000005, 62273.560000000005, 62273.562000000005, 62273.564, 62273.566, 62273.568, 62273.57, 62273.572, 62273.574, 62273.576, 62273.578, 62273.58, 62273.582, 62273.584, 62273.586], "Voltages"=[2.98, 2.98, 2.826, 2.672, 2.518, 2.364, 2.21, 2.056, 1.902, 1.748, 1.594, 1.44, 1.286, 1.1320000000000001, 0.9780000000000002, 0.8239999999999998, 0.6699999999999999, 0.516, 0.3620000000000001, 0.20800000000000018, 0.053999999999999826, -0.10000000000000009], "Enable Ch"=TRUE, "Hinge Points"=22}, {"Times"=[5500.0, 5600.0, 5609.0, 5618.0, 5627.0, 5636.0, 5645.0, 5654.0, 5663.0, 5672.0, 5681.0, 5690.0, 5699.0, 5708.0, 5717.0, 5726.0, 5735.0, 5744.0, 5753.0, 5762.0, 5771.0, 5780.0, 5789.0, 5798.0, 5807.0, 5816.0, 5825.0, 5834.0, 5843.0, 5852.0, 5861.0, 5870.0, 5879.0, 5888.0, 5897.0, 5906.0, 5915.0, 5924.0, 5933.0, 5942.0, 5951.0, 5960.0, 5969.0, 5978.0, 5987.0, 5996.0, 6005.0, 6014.0, 6023.0, 6032.0, 6041.0, 6050.0, 6059.0, 6068.0, 6077.0, 6086.0, 6095.0, 6104.0, 6113.0, 6122.0, 6131.0, 6140.0, 6149.0, 6158.0, 6167.0, 6176.0, 6185.0, 6194.0, 6203.0, 6212.0, 6221.0, 6230.0, 6239.0, 6248.0, 6257.0, 6266.0, 6275.0, 6284.0, 6293.0, 6302.0, 6311.0, 6320.0, 6329.0, 6338.0, 6347.0, 6356.0, 6365.0, 6374.0, 6383.0, 6392.0, 6401.0, 6410.0, 6419.0, 6428.0, 6437.0, 6446.0, 6455.0, 6464.0, 6473.0, 6482.0, 6491.0, 6500.0, 62273.546, 62303.546], "Voltages"=[0.5, 0.5, 0.5067, 0.5134, 0.5201, 0.5268, 0.5335, 0.5402, 0.5468999999999999, 0.5536, 0.5603, 0.567, 0.5737, 0.5804, 0.5871, 0.5938, 0.6005, 0.6072, 0.6139, 0.6206, 0.6273, 0.634, 0.6407, 0.6474, 0.6541, 0.6608, 0.6675, 0.6742, 0.6809, 0.6876, 0.6942999999999999, 0.701, 0.7077, 0.7143999999999999, 0.7211, 0.7278, 0.7344999999999999, 0.7412, 0.7479, 0.7545999999999999, 0.7613, 0.768, 0.7746999999999999, 0.7814, 0.7881, 0.7948, 0.8015, 0.8082, 0.8149, 0.8216, 0.8283, 0.835, 0.8416999999999999, 0.8484, 0.8551, 0.8617999999999999, 0.8684999999999999, 0.8752, 0.8818999999999999, 0.8886, 0.8953, 0.9019999999999999, 0.9087, 0.9154, 0.9220999999999999, 0.9288, 0.9355, 0.9421999999999999, 0.9489, 0.9556, 0.9622999999999999, 0.969, 0.9757, 0.9823999999999999, 0.9891, 0.9958, 1.0025, 1.0091999999999999, 1.0158999999999998, 1.0226, 1.0293, 1.036, 1.0427, 1.0493999999999999, 1.0560999999999998, 1.0628, 1.0695, 1.0762, 1.0829, 1.0896, 1.0962999999999998, 1.103, 1.1097, 1.1164, 1.1231, 1.1298, 1.1364999999999998, 1.1432, 1.1499, 1.1566, 1.1633, 1.17, -1.0, 0.0], "Enable Ch"=TRUE, "Hinge Points"=104}, {"Times"=[1000.6, 62283.546, 62295.546, 62783.546, 62795.546], "Voltages"=[1.3, -2.175, 0.0, -2.175, 0.0], "Enable Ch"=TRUE, "Hinge Points"=5}, {"Times"=[62283.546, 62783.546], "Voltages"=[-1.0, -1.0], "Enable Ch"=TRUE, "Hinge Points"=2}] {"Voltages" format="%.2f"; "Times" format="%.2f"}, 6 "Output":i32[][](array[numeric])=[[62794047, 3, 14, 0], [62794046, 3, 14, 1], [62793247, 3, 14, 0], [62793246, 3, 14, 1], [62788547, 3, 14, 0], [62788546, 3, 14, 1], [62794047, 3, 15, 0], [62794046, 3, 15, 1], [62791547, 3, 15, 0], [62791546, 3, 15, 1], [62795547, 3, 15, 0], [62795546, 3, 15, 1], [62783547, 3, 15, 0], [62783546, 3, 15, 1], [62783547, 3, 15, 0], [62783546, 3, 15, 1], [-1000, 0, 5, 0], [-1000, 0, 8, 0], [-1000, 0, 8, 0], [-1000, 0, 8, 0], [-1000, 0, 8, 1], [-1000, 0, 8, 1], [-1000, 0, 9, 0], [-1000, 0, 10, 0], [-1000, 0, 10, 0], [-1000, 0, 10, 1], [-1000, 0, 10, 1], [-1000, 0, 13, 0], [-1000, 0, 13, 0], [-1000, 0, 13, 1], [-1000, 0, 13, 1], [944000, 3, 14, 1], [944000, 3, 14, 1], [944000, 3, 14, 1], [944000, 3, 15, 1], [944000, 3, 15, 1], [944001, 3, 14, 0], [944001, 3, 14, 0], [944001, 3, 14, 0], [944001, 3, 15, 0], [944001, 3, 15, 0], [951100, 0, 6, 1], [951100, 1, 7, 1], [954000, 3, 14, 1], [954001, 3, 14, 0], [978100, 3, 15, 1], [978101, 3, 15, 0], [992000, 3, 14, 1], [992001, 3, 14, 0], [994000, 3, 14, 1], [994000, 3, 14, 1], [994000, 3, 14, 1], [994000, 3, 15, 1], [994000, 3, 15, 1], [994000, 3, 15, 1], [994001, 3, 14, 0], [994001, 3, 14, 0], [994001, 3, 14, 0], [994001, 3, 15, 0], [994001, 3, 15, 0], [994001, 3, 15, 0], [998300, 0, 2, 0], [998300, 0, 4, 0], [998400, 0, 8, 1], [998400, 0, 9, 1], [999000, 0, 3, 0], [999100, 1, 9, 1], [1000000, 0, 10, 0], [1000000, 1, 0, 0], [1000000, 3, 14, 1], [1000000, 3, 14, 1], [1000000, 3, 14, 1], [1000000, 3, 15, 1], [1000001, 3, 14, 0], [1000001, 3, 14, 0], [1000001, 3, 14, 0], [1000001, 3, 15, 0], [1000100, 3, 14, 1], [1000100, 3, 15, 1], [1000101, 3, 14, 0], [1000101, 3, 15, 0], [1000600, 3, 14, 1], [1000600, 3, 14, 1], [1000600, 3, 15, 1], [1000600, 3, 15, 1], [1000601, 3, 14, 0], [1000601, 3, 14, 0], [1000601, 3, 15, 0], [1000601, 3, 15, 0], [1001000, 3, 15, 1], [1001000, 3, 15, 1], [1001001, 3, 15, 0], [1001001, 3, 15, 0], [1001100, 0, 5, 1], [1001100, 0, 10, 1], [1001100, 1, 1, 1], [1002100, 1, 1, 0], [1002100, 1, 9, 0], [1002600, 0, 5, 0], [1003100, 0, 8, 0], [1003100, 0, 9, 0], [1003100, 1, 0, 1], [1003100, 3, 15, 1], [1003101, 3, 15, 0], [1004100, 0, 6, 0], [1004100, 0, 10, 0], [1004100, 1, 7, 0], [1004100, 3, 15, 1], [1004101, 3, 15, 0], [1008100, 3, 15, 1], [1008101, 3, 15, 0], [1011100, 3, 14, 1], [1011101, 3, 14, 0], [1183100, 3, 15, 1], [1183101, 3, 15, 0], [1188100, 3, 15, 1], [1188101, 3, 15, 0], [1193100, 3, 15, 1], [1193101, 3, 15, 0], [1198100, 3, 15, 1], [1198101, 3, 15, 0], [1203100, 3, 15, 1], [1203100, 3, 15, 1], [1203101, 3, 15, 0], [1203101, 3, 15, 0], [1208100, 3, 15, 1], [1208100, 3, 15, 1], [1208101, 3, 15, 0], [1208101, 3, 15, 0], [1213100, 3, 15, 1], [1213100, 3, 15, 1], [1213101, 3, 15, 0], [1213101, 3, 15, 0], [1218100, 3, 15, 1], [1218100, 3, 15, 1], [1218101, 3, 15, 0], [1218101, 3, 15, 0], [1223100, 3, 15, 1], [1223100, 3, 15, 1], [1223101, 3, 15, 0], [1223101, 3, 15, 0], [1228100, 3, 15, 1], [1228100, 3, 15, 1], [1228101, 3, 15, 0], [1228101, 3, 15, 0], [1233100, 3, 15, 1], [1233100, 3, 15, 1], [1233101, 3, 15, 0], [1233101, 3, 15, 0], [1238100, 3, 15, 1], [1238100, 3, 15, 1], [1238101, 3, 15, 0], [1238101, 3, 15, 0], [1243100, 3, 15, 1], [1243100, 3, 15, 1], [1243101, 3, 15, 0], [1243101, 3, 15, 0], [1248100, 3, 15, 1], [1248100, 3, 15, 1], [1248101, 3, 15, 0], [1248101, 3, 15, 0], [1253100, 3, 15, 1], [1253100, 3, 15, 1], [1253101, 3, 15, 0], [1253101, 3, 15, 0], [1258100, 3, 15, 1], [1258100, 3, 15, 1], [1258101, 3, 15, 0], [1258101, 3, 15, 0], [1263100, 3, 15, 1], [1263100, 3, 15, 1], [1263101, 3, 15, 0], [1263101, 3, 15, 0], [1268100, 3, 15, 1], [1268100, 3, 15, 1], [1268101, 3, 15, 0], [1268101, 3, 15, 0], [1273100, 3, 15, 1], [1273100, 3, 15, 1], [1273101, 3, 15, 0], [1273101, 3, 15, 0], [1278100, 3, 15, 1], [1278100, 3, 15, 1], [1278101, 3, 15, 0], [1278101, 3, 15, 0], [1283100, 3, 15, 1], [1283100, 3, 15, 1], [1283101, 3, 15, 0], [1283101, 3, 15, 0], [1288100, 3, 15, 1], [1288100, 3, 15, 1], [1288101, 3, 15, 0], [1288101, 3, 15, 0], [1293100, 3, 15, 1], [1293100, 3, 15, 1], [1293101, 3, 15, 0], [1293101, 3, 15, 0], [1298100, 3, 15, 1], [1298100, 3, 15, 1], [1298101, 3, 15, 0], [1298101, 3, 15, 0], [1303100, 3, 15, 1], [1303100, 3, 15, 1], [1303101, 3, 15, 0], [1303101, 3, 15, 0], [1308100, 3, 15, 1], [1308100, 3, 15, 1], [1308101, 3, 15, 0], [1308101, 3, 15, 0], [1313100, 3, 15, 1], [1313100, 3, 15, 1], [1313101, 3, 15, 0], [1313101, 3, 15, 0], [1318100, 3, 15, 1], [1318100, 3, 15, 1], [1318101, 3, 15, 0], [1318101, 3, 15, 0], [1323100, 3, 15, 1], [1323100, 3, 15, 1], [1323101, 3, 15, 0], [1323101, 3, 15, 0], [1328100, 3, 15, 1], [1328100, 3, 15, 1], [1328101, 3, 15, 0], [1328101, 3, 15, 0], [1333100, 3, 15, 1], [1333100, 3, 15, 1], [1333101, 3, 15, 0], [1333101, 3, 15, 0], [1338100, 3, 15, 1], [1338100, 3, 15, 1], [1338101, 3, 15, 0], [1338101, 3, 15, 0], [1343100, 3, 15, 1], [1343100, 3, 15, 1], [1343101, 3, 15, 0], [1343101, 3, 15, 0], [1348100, 3, 15, 1], [1348100, 3, 15, 1], [1348101, 3, 15, 0], [1348101, 3, 15, 0], [1353100, 3, 15, 1], [1353100, 3, 15, 1], [1353101, 3, 15, 0], [1353101, 3, 15, 0], [1358100, 3, 15, 1], [1358100, 3, 15, 1], [1358101, 3, 15, 0], [1358101, 3, 15, 0], [1363100, 3, 15, 1], [1363100, 3, 15, 1], [1363101, 3, 15, 0], [1363101, 3, 15, 0], [1368100, 3, 15, 1], [1368100, 3, 15, 1], [1368101, 3, 15, 0], [1368101, 3, 15, 0], [1373100, 3, 15, 1], [1373100, 3, 15, 1], [1373101, 3, 15, 0], [1373101, 3, 15, 0], [1378100, 3, 15, 1], [1378100, 3, 15, 1], [1378101, 3, 15, 0], [1378101, 3, 15, 0], [1383100, 3, 15, 1], [1383100, 3, 15, 1], [1383101, 3, 15, 0], [1383101, 3, 15, 0], [1388100, 3, 15, 1], [1388100, 3, 15, 1], [1388101, 3, 15, 0], [1388101, 3, 15, 0], [1393100, 3, 15, 1], [1393100, 3, 15, 1], [1393101, 3, 15, 0], [1393101, 3, 15, 0], [1398100, 3, 15, 1], [1398100, 3, 15, 1], [1398101, 3, 15, 0], [1398101, 3, 15, 0], [1403100, 3, 15, 1], [1403100, 3, 15, 1], [1403101, 3, 15, 0], [1403101, 3, 15, 0], [1408100, 3, 15, 1], [1408100, 3, 15, 1], [1408101, 3, 15, 0], [1408101, 3, 15, 0], [1413100, 3, 15, 1], [1413100, 3, 15, 1], [1413101, 3, 15, 0], [1413101, 3, 15, 0], [1418100, 3, 15, 1], [1418100, 3, 15, 1], [1418101, 3, 15, 0], [1418101, 3, 15, 0], [1423100, 3, 15, 1], [1423100, 3, 15, 1], [1423101, 3, 15, 0], [1423101, 3, 15, 0], [1428100, 3, 15, 1], [1428100, 3, 15, 1], [1428101, 3, 15, 0], [1428101, 3, 15, 0], [1433100, 3, 15, 1], [1433100, 3, 15, 1], [1433101, 3, 15, 0], [1433101, 3, 15, 0], [1438100, 3, 15, 1], [1438100, 3, 15, 1], [1438101, 3, 15, 0], [1438101, 3, 15, 0], [1443100, 3, 15, 1], [1443100, 3, 15, 1], [1443101, 3, 15, 0], [1443101, 3, 15, 0], [1448100, 3, 15, 1], [1448100, 3, 15, 1], [1448101, 3, 15, 0], [1448101, 3, 15, 0], [1453100, 3, 15, 1], [1453100, 3, 15, 1], [1453101, 3, 15, 0], [1453101, 3, 15, 0], [1458100, 3, 15, 1], [1458100, 3, 15, 1], [1458101, 3, 15, 0], [1458101, 3, 15, 0], [1463100, 3, 15, 1], [1463100, 3, 15, 1], [1463101, 3, 15, 0], [1463101, 3, 15, 0], [1468100, 3, 15, 1], [1468100, 3, 15, 1], [1468101, 3, 15, 0], [1468101, 3, 15, 0], [1473100, 3, 15, 1], [1473100, 3, 15, 1], [1473101, 3, 15, 0], [1473101, 3, 15, 0], [1478100, 3, 15, 1], [1478100, 3, 15, 1], [1478101, 3, 15, 0], [1478101, 3, 15, 0], [1483100, 3, 15, 1], [1483100, 3, 15, 1], [1483101, 3, 15, 0], [1483101, 3, 15, 0], [1488100, 3, 15, 1], [1488100, 3, 15, 1], [1488101, 3, 15, 0], [1488101, 3, 15, 0], [1493100, 3, 15, 1], [1493100, 3, 15, 1], [1493101, 3, 15, 0], [1493101, 3, 15, 0], [1498100, 3, 15, 1], [1498100, 3, 15, 1], [1498101, 3, 15, 0], [1498101, 3, 15, 0], [1500000, 1, 3, 1], [1503100, 3, 15, 1], [1503100, 3, 15, 1], [1503101, 3, 15, 0], [1503101, 3, 15, 0], [1508100, 3, 15, 1], [1508100, 3, 15, 1], [1508101, 3, 15, 0], [1508101, 3, 15, 0], [1513100, 3, 15, 1], [1513100, 3, 15, 1], [1513101, 3, 15, 0], [1513101, 3, 15, 0], [1518100, 3, 15, 1], [1518100, 3, 15, 1], [1518101, 3, 15, 0], [1518101, 3, 15, 0], [1523100, 3, 15, 1], [1523100, 3, 15, 1], [1523101, 3, 15, 0], [1523101, 3, 15, 0], [1528100, 3, 15, 1], [1528100, 3, 15, 1], [1528101, 3, 15, 0], [1528101, 3, 15, 0], [1533100, 3, 15, 1], [1533100, 3, 15, 1], [1533101, 3, 15, 0], [1533101, 3, 15, 0], [1538100, 3, 15, 1], [1538100, 3, 15, 1], [1538101, 3, 15, 0], [1538101, 3, 15, 0], [1543100, 3, 15, 1], [1543100, 3, 15, 1], [1543101, 3, 15, 0], [1543101, 3, 15, 0], [1548100, 3, 15, 1], [1548100, 3, 15, 1], [1548101, 3, 15, 0], [1548101, 3, 15, 0], [1553100, 3, 15, 1], [1553100, 3, 15, 1], [1553101, 3, 15, 0], [1553101, 3, 15, 0], [1558100, 3, 15, 1], [1558100, 3, 15, 1], [1558101, 3, 15, 0], [1558101, 3, 15, 0], [1563100, 3, 15, 1], [1563100, 3, 15, 1], [1563101, 3, 15, 0], [1563101, 3, 15, 0], [1568100, 3, 15, 1], [1568100, 3, 15, 1], [1568101, 3, 15, 0], [1568101, 3, 15, 0], [1573100, 3, 15, 1], [1573100, 3, 15, 1], [1573101, 3, 15, 0], [1573101, 3, 15, 0], [1578100, 3, 15, 1], [1578100, 3, 15, 1], [1578101, 3, 15, 0], [1578101, 3, 15, 0], [1583100, 3, 15, 1], [1583100, 3, 15, 1], [1583101, 3, 15, 0], [1583101, 3, 15, 0], [1588100, 3, 15, 1], [1588100, 3, 15, 1], [1588101, 3, 15, 0], [1588101, 3, 15, 0], [1593100, 3, 15, 1], [1593100, 3, 15, 1], [1593101, 3, 15, 0], [1593101, 3, 15, 0], [1598100, 3, 15, 1], [1598100, 3, 15, 1], [1598101, 3, 15, 0], [1598101, 3, 15, 0], [1603100, 3, 15, 1], [1603100, 3, 15, 1], [1603101, 3, 15, 0], [1603101, 3, 15, 0], [1608100, 3, 15, 1], [1608100, 3, 15, 1], [1608101, 3, 15, 0], [1608101, 3, 15, 0], [1613100, 3, 15, 1], [1613100, 3, 15, 1], [1613101, 3, 15, 0], [1613101, 3, 15, 0], [1618100, 3, 15, 1], [1618100, 3, 15, 1], [1618101, 3, 15, 0], [1618101, 3, 15, 0], [1623100, 3, 15, 1], [1623100, 3, 15, 1], [1623101, 3, 15, 0], [1623101, 3, 15, 0], [1628100, 3, 15, 1], [1628100, 3, 15, 1], [1628101, 3, 15, 0], [1628101, 3, 15, 0], [1633100, 3, 15, 1], [1633100, 3, 15, 1], [1633101, 3, 15, 0], [1633101, 3, 15, 0], [1638100, 3, 15, 1], [1638100, 3, 15, 1], [1638101, 3, 15, 0], [1638101, 3, 15, 0], [1643100, 3, 15, 1], [1643100, 3, 15, 1], [1643101, 3, 15, 0], [1643101, 3, 15, 0], [1648100, 3, 15, 1], [1648100, 3, 15, 1], [1648101, 3, 15, 0], [1648101, 3, 15, 0], [1653100, 3, 15, 1], [1653100, 3, 15, 1], [1653101, 3, 15, 0], [1653101, 3, 15, 0], [1658100, 3, 15, 1], [1658100, 3, 15, 1], [1658101, 3, 15, 0], [1658101, 3, 15, 0], [1663100, 3, 15, 1], [1663100, 3, 15, 1], [1663101, 3, 15, 0], [1663101, 3, 15, 0], [1668100, 3, 15, 1], [1668100, 3, 15, 1], [1668101, 3, 15, 0], [1668101, 3, 15, 0], [1673100, 3, 15, 1], [1673100, 3, 15, 1], [1673101, 3, 15, 0], [1673101, 3, 15, 0], [1678100, 3, 15, 1], [1678100, 3, 15, 1], [1678101, 3, 15, 0], [1678101, 3, 15, 0], [1683100, 3, 15, 1], [1683100, 3, 15, 1], [1683101, 3, 15, 0], [1683101, 3, 15, 0], [1688100, 3, 15, 1], [1688101, 3, 15, 0], [1693100, 3, 15, 1], [1693101, 3, 15, 0], [1698100, 3, 15, 1], [1698101, 3, 15, 0], [1703100, 3, 15, 1], [1703101, 3, 15, 0], [5499900, 3, 15, 1], [5499901, 3, 15, 0], [5500000, 1, 14, 1], [5500000, 1, 15, 1], [5500000, 3, 15, 1], [5500000, 3, 15, 1], [5500001, 3, 15, 0], [5500001, 3, 15, 0], [5505000, 3, 15, 1], [5505001, 3, 15, 0], [5600000, 3, 15, 1], [5600001, 3, 15, 0], [5609000, 3, 15, 1], [5609001, 3, 15, 0], [5618000, 3, 15, 1], [5618001, 3, 15, 0], [5627000, 3, 15, 1], [5627001, 3, 15, 0], [5636000, 3, 15, 1], [5636001, 3, 15, 0], [5645000, 3, 15, 1], [5645001, 3, 15, 0], [5654000, 3, 15, 1], [5654001, 3, 15, 0], [5663000, 3, 15, 1], [5663001, 3, 15, 0], [5672000, 3, 15, 1], [5672001, 3, 15, 0], [5681000, 3, 15, 1], [5681001, 3, 15, 0], [5690000, 3, 15, 1], [5690001, 3, 15, 0], [5699000, 3, 15, 1], [5699001, 3, 15, 0], [5708000, 3, 15, 1], [5708001, 3, 15, 0], [5717000, 3, 15, 1], [5717001, 3, 15, 0], [5726000, 3, 15, 1], [5726001, 3, 15, 0], [5735000, 3, 15, 1], [5735001, 3, 15, 0], [5744000, 3, 15, 1], [5744001, 3, 15, 0], [5753000, 3, 15, 1], [5753001, 3, 15, 0], [5762000, 3, 15, 1], [5762001, 3, 15, 0], [5771000, 3, 15, 1], [5771001, 3, 15, 0], [5780000, 3, 15, 1], [5780001, 3, 15, 0], [5789000, 3, 15, 1], [5789001, 3, 15, 0], [5798000, 3, 15, 1], [5798001, 3, 15, 0], [5807000, 3, 15, 1], [5807001, 3, 15, 0], [5816000, 3, 15, 1], [5816001, 3, 15, 0], [5825000, 3, 15, 1], [5825001, 3, 15, 0], [5834000, 3, 15, 1], [5834001, 3, 15, 0], [5843000, 3, 15, 1], [5843001, 3, 15, 0], [5852000, 3, 15, 1], [5852001, 3, 15, 0], [5861000, 3, 15, 1], [5861001, 3, 15, 0], [5870000, 3, 15, 1], [5870001, 3, 15, 0], [5879000, 3, 15, 1], [5879001, 3, 15, 0], [5888000, 3, 15, 1], [5888001, 3, 15, 0], [5897000, 3, 15, 1], [5897001, 3, 15, 0], [5906000, 3, 15, 1], [5906001, 3, 15, 0], [5915000, 3, 15, 1], [5915001, 3, 15, 0], [5924000, 3, 15, 1], [5924001, 3, 15, 0], [5933000, 3, 15, 1], [5933001, 3, 15, 0], [5942000, 3, 15, 1], [5942001, 3, 15, 0], [5951000, 3, 15, 1], [5951001, 3, 15, 0], [5960000, 3, 15, 1], [5960001, 3, 15, 0], [5969000, 3, 15, 1], [5969001, 3, 15, 0], [5978000, 3, 15, 1], [5978001, 3, 15, 0], [5987000, 3, 15, 1], [5987001, 3, 15, 0], [5996000, 3, 15, 1], [5996001, 3, 15, 0], [6005000, 3, 15, 1], [6005001, 3, 15, 0], [6014000, 3, 15, 1], [6014001, 3, 15, 0], [6023000, 3, 15, 1], [6023001, 3, 15, 0], [6032000, 3, 15, 1], [6032001, 3, 15, 0], [6041000, 3, 15, 1], [6041001, 3, 15, 0], [6050000, 3, 15, 1], [6050001, 3, 15, 0], [6059000, 3, 15, 1], [6059001, 3, 15, 0], [6068000, 3, 15, 1], [6068001, 3, 15, 0], [6077000, 3, 15, 1], [6077001, 3, 15, 0], [6086000, 3, 15, 1], [6086001, 3, 15, 0], [6095000, 3, 15, 1], [6095001, 3, 15, 0], [6104000, 3, 15, 1], [6104001, 3, 15, 0], [6113000, 3, 15, 1], [6113001, 3, 15, 0], [6122000, 3, 15, 1], [6122001, 3, 15, 0], [6131000, 3, 15, 1], [6131001, 3, 15, 0], [6140000, 3, 15, 1], [6140001, 3, 15, 0], [6149000, 3, 15, 1], [6149001, 3, 15, 0], [6158000, 3, 15, 1], [6158001, 3, 15, 0], [6167000, 3, 15, 1], [6167001, 3, 15, 0], [6176000, 3, 15, 1], [6176001, 3, 15, 0], [6185000, 3, 15, 1], [6185001, 3, 15, 0], [6194000, 3, 15, 1], [6194001, 3, 15, 0], [6203000, 3, 15, 1], [6203001, 3, 15, 0], [6212000, 3, 15, 1], [6212001, 3, 15, 0], [6221000, 3, 15, 1], [6221001, 3, 15, 0], [6230000, 3, 15, 1], [6230001, 3, 15, 0], [6239000, 3, 15, 1], [6239001, 3, 15, 0], [6248000, 3, 15, 1], [6248001, 3, 15, 0], [6257000, 3, 15, 1], [6257001, 3, 15, 0], [6266000, 3, 15, 1], [6266001, 3, 15, 0], [6275000, 3, 15, 1], [6275001, 3, 15, 0], [6284000, 3, 15, 1], [6284001, 3, 15, 0], [6293000, 3, 15, 1], [6293001, 3, 15, 0], [6302000, 3, 15, 1], [6302001, 3, 15, 0], [6311000, 3, 15, 1], [6311001, 3, 15, 0], [6320000, 3, 15, 1], [6320001, 3, 15, 0], [6329000, 3, 15, 1], [6329001, 3, 15, 0], [6338000, 3, 15, 1], [6338001, 3, 15, 0], [6347000, 3, 15, 1], [6347001, 3, 15, 0], [6356000, 3, 15, 1], [6356001, 3, 15, 0], [6365000, 3, 15, 1], [6365001, 3, 15, 0], [6374000, 3, 15, 1], [6374001, 3, 15, 0], [6383000, 3, 15, 1], [6383001, 3, 15, 0], [6392000, 3, 15, 1], [6392001, 3, 15, 0], [6401000, 3, 15, 1], [6401001, 3, 15, 0], [6410000, 3, 15, 1], [6410001, 3, 15, 0], [6419000, 3, 15, 1], [6419001, 3, 15, 0], [6428000, 3, 15, 1], [6428001, 3, 15, 0], [6437000, 3, 15, 1], [6437001, 3, 15, 0], [6446000, 3, 15, 1], [6446001, 3, 15, 0], [6455000, 3, 15, 1], [6455001, 3, 15, 0], [6464000, 3, 15, 1], [6464001, 3, 15, 0], [6473000, 3, 15, 1], [6473001, 3, 15, 0], [6482000, 3, 15, 1], [6482001, 3, 15, 0], [6491000, 3, 15, 1], [6491001, 3, 15, 0], [6500000, 3, 14, 1], [6500000, 3, 15, 1], [6500000, 3, 15, 1], [6500001, 3, 14, 0], [6500001, 3, 15, 0], [6500001, 3, 15, 0], [7500000, 1, 0, 0], [7500000, 1, 3, 0], [62173546, 1, 14, 0], [62223546, 1, 8, 1], [62272746, 1, 9, 1], [62273546, 3, 15, 1], [62273546, 3, 15, 1], [62273546, 3, 15, 1], [62273547, 3, 15, 0], [62273547, 3, 15, 0], [62273547, 3, 15, 0], [62273548, 3, 15, 1], [62273549, 3, 15, 0], [62273550, 3, 15, 1], [62273551, 3, 15, 0], [62273552, 3, 15, 1], [62273553, 3, 15, 0], [62273554, 3, 15, 1], [62273555, 3, 15, 0], [62273556, 3, 15, 1], [62273557, 3, 15, 0], [62273558, 3, 15, 1], [62273559, 3, 15, 0], [62273560, 3, 15, 1], [62273561, 3, 15, 0], [62273562, 3, 15, 1], [62273563, 3, 15, 0], [62273564, 3, 15, 1], [62273565, 3, 15, 0], [62273566, 3, 15, 1], [62273567, 3, 15, 0], [62273568, 3, 15, 1], [62273569, 3, 15, 0], [62273570, 3, 15, 1], [62273571, 3, 15, 0], [62273572, 3, 15, 1], [62273573, 3, 15, 0], [62273574, 3, 15, 1], [62273575, 3, 15, 0], [62273576, 3, 15, 1], [62273577, 3, 15, 0], [62273578, 3, 15, 1], [62273579, 3, 15, 0], [62273580, 3, 15, 1], [62273581, 3, 15, 0], [62273582, 3, 15, 1], [62273583, 3, 15, 0], [62273584, 3, 15, 1], [62273585, 3, 15, 0], [62273586, 3, 15, 1], [62273587, 3, 15, 0], [62283546, 3, 15, 1], [62283546, 3, 15, 1], [62283547, 3, 15, 0], [62283547, 3, 15, 0], [62287546, 0, 1, 1], [62288546, 3, 14, 1], [62288547, 3, 14, 0], [62289546, 0, 7, 1], [62290546, 1, 14, 1], [62291546, 3, 15, 1], [62291547, 3, 15, 0], [62293246, 3, 14, 1], [62293247, 3, 14, 0], [62293346, 0, 12, 1], [62293446, 1, 7, 1], [62293546, 0, 1, 0], [62293546, 0, 12, 0], [62293546, 0, 15, 1], [62293546, 1, 1, 1], [62293646, 0, 7, 0], [62293646, 0, 15, 0], [62293646, 1, 1, 0], [62293646, 1, 7, 0], [62293646, 1, 14, 0], [62294046, 3, 14, 1], [62294046, 3, 15, 1], [62294047, 3, 14, 0], [62294047, 3, 15, 0], [62295546, 3, 15, 1], [62295547, 3, 15, 0], [62303546, 3, 15, 1], [62303547, 3, 15, 0], [62323546, 1, 9, 0], [62373546, 1, 15, 0], [62789546, 0, 7, 1], [62790546, 1, 14, 1], [62793346, 0, 12, 1], [62793446, 1, 7, 1], [62793546, 0, 12, 0], [62793546, 0, 15, 1], [62793546, 1, 1, 1], [62793646, 0, 7, 0], [62793646, 0, 15, 0], [62793646, 1, 1, 0], [62793646, 1, 7, 0], [62793646, 1, 14, 0]], 7 "GPIB Output":T1(array[cluster]) {"Module" items=["TTL high                                                                                 ", "TTL low                          ", "Camera Strobe                   ", "CMOT", "Defaults                           ", "Fluorescence pulse           ", "IP trap                         ", "Kinetics OD image          ", "Kinetics picture", "Kinetics probe pulse", "MOT light only                ", "MOT off                                   ", "MOT on                         ", "Move cart                      ", "OD image                     ", "Optical pumping          ", "Picture                             ", "Probe Pulse", "Quadrupole trap             ", "IP off", "Utility Module 02           ", "Utility Module 03           ", "Molasses          ", "Utility Module 04     ", "Utility Module 05     ", "Utility Module 06     ", "Utility Module 07     ", "Utility Module 08     ", "Utility Module 09     ", "Utility Module 10     ", "Static DAC", "GPIB"]; "Abs Start Time" format="%.3f"})   [LabVIEW 2015]
panel:
  in  "Read/Write":bool
  in  "Do Write/Read":bool
  in  "Manual Array":T2(array[cluster])=[{"Time2 (ms)"=-10.0, "Port2"=4, "Line2"=15, "Comments2"="Rb Probe Detuning", "Value2"=FALSE, "Enable2"=TRUE, "DAC value"=-1.0}, {"Time2 (ms)"=-10.0, "Port2"=4, "Line2"=14, "Comments2"="Rb Probe Power", "Value2"=FALSE, "Enable2"=TRUE, "DAC value"=-2.175}, {"Time2 (ms)"=-4.0, "Port2"=0, "Line2"=7, "Comments2"="Rb F =2 probe shutter on", "Value2"=TRUE, "Enable2"=TRUE, "DAC value"=0.0}, {"Time2 (ms)"=0.0, "Port2"=1, "Line2"=1, "Comments2"="Rb AOM Probe On", "Value2"=TRUE, "Enable2"=TRUE, "DAC value"=0.0}, {"Time2 (ms)"=0.1, "Port2"=1, "Line2"=1, "Comments2"="Rb AOM Probe Off", "Value2"=FALSE, "Enable2"=TRUE, "DAC value"=0.0}, {"Time2 (ms)"=0.1, "Port2"=0, "Line2"=7, "Comments2"="Rb F =2 probe shutter off", "Value2"=FALSE, "Enable2"=TRUE, "DAC value"=0.0}, {"Time2 (ms)"=2.0, "Port2"=4, "Line2"=14, "Comments2"="Rb Probe Power off", "Value2"=FALSE, "Enable2"=TRUE, "DAC value"=0.0}, {"Time2 (ms)"=-2.0, "Port2"=4, "Line2"=11, "Comments2"="Rb Repump Power", "Value2"=FALSE, "Enable2"=TRUE, "DAC value"=-0.4}, {"Time2 (ms)"=-2.5, "Port2"=0, "Line2"=8, "Comments2"="Rb Repump Shutter On", "Value2"=TRUE, "Enable2"=FALSE, "DAC value"=0.0}, {"Time2 (ms)"=-0.1, "Port2"=1, "Line2"=7, "Comments2"="Rb Repump AOM on for imaging", "Value2"=TRUE, "Enable2"=TRUE, "DAC value"=0.0}, {"Time2 (ms)"=0.1, "Port2"=1, "Line2"=7, "Comments2"="Rb Repump AOM off for imaging", "Value2"=FALSE, "Enable2"=TRUE, "DAC value"=0.0}, {"Time2 (ms)"=1.0, "Port2"=0, "Line2"=8, "Comments2"="Rb Repump Shutter Off", "Value2"=FALSE, "Enable2"=FALSE, "DAC value"=0.0}, {"Time2 (ms)"=0.5, "Port2"=4, "Line2"=11, "Comments2"="Rb Repump Power off", "Value2"=FALSE, "Enable2"=TRUE, "DAC value"=0.0}, {"Time2 (ms)"=-5.0, "Port2"=4, "Line2"=7, "Comments2"="Na Probe Detuning", "Value2"=FALSE, "Enable2"=TRUE, "DAC value"=0.0}, {"Time2 (ms)"=-3.0, "Port2"=1, "Line2"=14, "Comments2"="Na probe shutter on", "Value2"=TRUE, "Enable2"=TRUE, "DAC value"=0.0}, {"Time2 (ms)"=0.0, "Port2"=0, "Line2"=15, "Comments2"="Na AOM probe on", "Value2"=TRUE, "Enable2"=TRUE, "DAC value"=0.0}, {"Time2 (ms)"=0.1, "Port2"=0, "Line2"=15, "Comments2"="Na AOM Probe off", "Value2"=FALSE, "Enable2"=TRUE, "DAC value"=0.0}, {"Time2 (ms)"=0.1, "Port2"=1, "Line2"=14, "Comments2"="Na probe shutter off", "Value2"=FALSE, "Enable2"=TRUE, "DAC value"=0.0}, {"Time2 (ms)"=-0.3, "Port2"=4, "Line2"=4, "Comments2"="Na Repump Power", "Value2"=FALSE, "Enable2"=TRUE, "DAC value"=-0.8}, {"Time2 (ms)"=-3.0, "Port2"=0, "Line2"=10, "Comments2"="Na Repump Shutter On", "Value2"=TRUE, "Enable2"=FALSE, "DAC value"=0.0}, {"Time2 (ms)"=-3.0, "Port2"=0, "Line2"=13, "Comments2"="Na 3rd Repump Shutter On (imaging for Dark MOT)", "Value2"=TRUE, "Enable2"=FALSE, "DAC value"=0.0}, {"Time2 (ms)"=-0.2, "Port2"=0, "Line2"=12, "Comments2"="Na Repump AOM on for imaging", "Value2"=TRUE, "Enable2"=TRUE, "DAC value"=0.0}, {"Time2 (ms)"=0.0, "Port2"=0, "Line2"=12, "Comments2"="Na Repump AOM off for imaging", "Value2"=FALSE, "Enable2"=TRUE, "DAC value"=0.0}, {"Time2 (ms)"=0.1, "Port2"=0, "Line2"=13, "Comments2"="Na 3rd Repump Shutter off (imaging for Dark MOT)", "Value2"=FALSE, "Enable2"=FALSE, "DAC value"=0.0}, {"Time2 (ms)"=0.1, "Port2"=0, "Line2"=10, "Comments2"="Na Repump Shutter Off", "Value2"=FALSE, "Enable2"=FALSE, "DAC value"=0.0}, {"Time2 (ms)"=0.5, "Port2"=4, "Line2"=4, "Comments2"="Na Repump Power Off", "Value2"=FALSE, "Enable2"=TRUE, "DAC value"=0.0}] {"Line2" items=["0", "1", "2", "3", "4", "5", "6", "7", "8", "9", "10", "11", "12", "13", "14", "15"]; "Port2" items=["A", "B", "C", "D", "DAC", "GPIB"]; "Time2 (ms)" format="%.3f"}
  in  "filename":string="probe pulse"
  in  "Static DAC Linear Ramps":T3(array[cluster]) {"end value" format="%_6g"; "start value" format="%_6g"; "Ramp end" format="%_6g"; "Ramp begin" format="%_6g"; "DAC Channel" items=["0", "1", "2", "3", "4", "5", "6", "7", "8", "9", "10", "11", "12", "13", "14", "0"]}
  # "Time                   Port        Line       Value  Enable  DAC voltage  Comments"
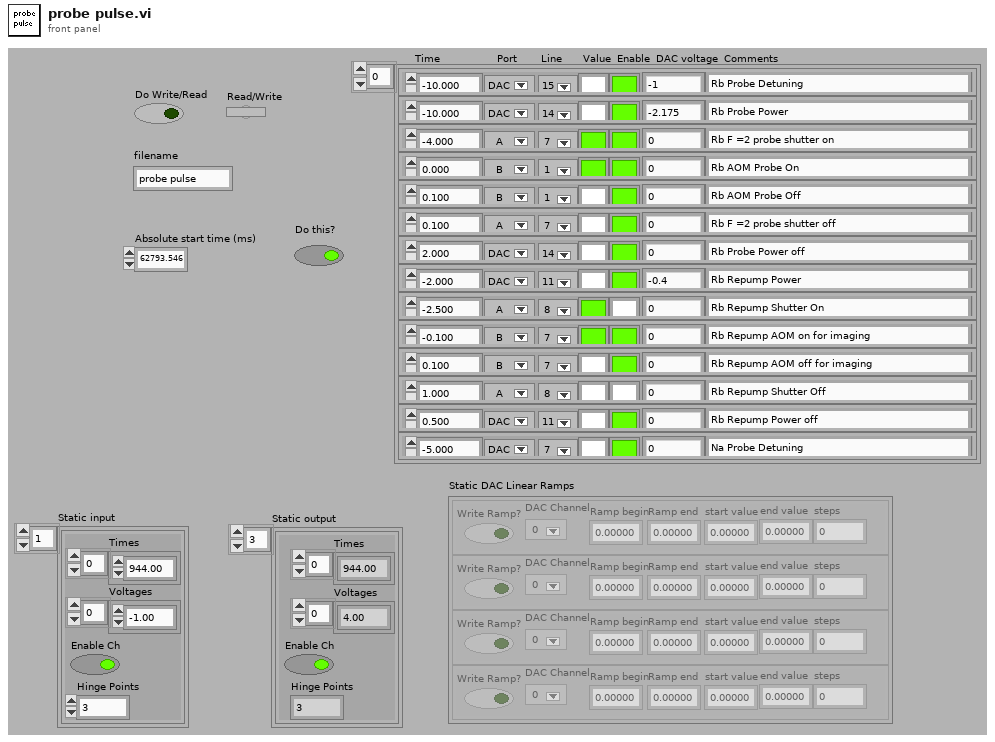
[diagram p1: front panel]
types:
  T1 = cluster{"Enable":bool, "Abs Start Time":dbl, "Module":u16, "String":string, "Array":string[]}[]
  T2 = cluster{"Time2 (ms)":dbl, "Port2":u16, "Line2":u16, "Comments2":string, "Value2":bool, "Enable2":bool, "DAC value":dbl}[]
  T3 = cluster{"Write Ramp?":bool, "DAC Channel":i16, "Ramp begin":dbl, "Ramp end":dbl, "start value":dbl, "end value":dbl, "steps":i16}[]
  T4 = cluster{"Times":dbl[], "Voltages":dbl[], "Enable Ch":bool, "Hinge Points":u8}[]
  T5 = cluster{"Manual Array":cluster{"Time2 (ms)":dbl, "Port2":u16, "Line2":u16, "Comments2":string, "Value2":bool, "Enable2":bool, "DAC value":dbl}[], "Static DAC Linear Ramps":cluster{"Write Ramp?":bool, "DAC Channel":i16, "Ramp begin":dbl, "Ramp end":dbl, "start value":dbl, "end value":dbl, "steps":i16}[]}
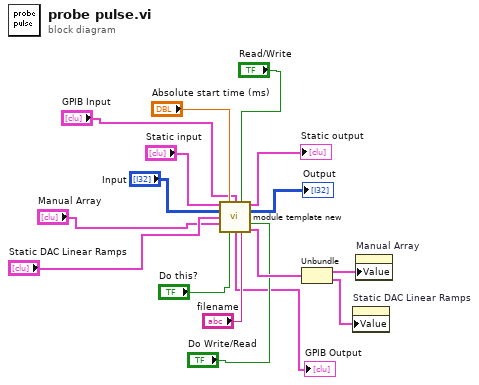
[diagram p0: block diagram]
diagram:
  n1 = call "module template new.vi"("Static input"="Static input", "Absolute start time (ms)"="Absolute start time (ms)", "GPIB Input"="GPIB Input", "Read/Write"="Read/Write", "Input"="Input", "Static DAC Linear Ramps"="Static DAC Linear Ramps", "Manual Array"="Manual Array", "Do Write/Read"="Do Write/Read", "Do this?"="Do this?", "filename"="filename") -> ("Static output"=→"Static output":T4, "Output"=→"Output":i32[][], "GPIB Output"=→"GPIB Output":T1, "Saved Cluster"=w5:T5)  [unwired: 2 in]
  n2 = Unbundle(w5) -> ("Manual Array"=w7:T2, "Static DAC Linear Ramps"=w6:T3)
  n3 = property on="Static DAC Linear Ramps" class="Arr (strict)"("Value"=w6) -> ()  [unwired: 2 in, 2 out]
  n4 = property on="Manual Array" class="Arr (strict)"("Value"=w7) -> ()  [unwired: 2 in, 2 out]
